vi "XLP80_Action_InitControls.vi"(8 "err in":errorcluster) -> (0 "err out":errorcluster)   [LabVIEW 2021]
uses:
  XLP80_General_Libs/WL_Libs_V14.25/WL_Alarm_V14.00.llb/WL_Alarm_TypeDefClusterStatus.ctl
  XLP80_GUI_V001.llb/XLP80_GUI_TDefEnumMessages.ctl
  XLP80_HH/XLP80_HH_TDefsCluster_HH Setpoint.ctl
  XLP80_Globals/Globals_Settings_XLP80.vi
  XLP80_Globals/XLP80_Globals_Status.vi
  XLP80_Globals/XLP80_Globals_Referenzen.vi
  XLP80_Datalog/XLP80_Datalog_Globals.vi
  XLP80_Alarm_V001.llb/XLP80_Alarm_Globals.vi
  XLP80_HH/XLP80_HH_Globals.vi
  XLP80_General_Libs/WL_Libs_V14.25/WL_Alarm_V14.00.llb/WL_Alarm_Globals.vi
  XLP80_Auto_V001.llb/XLP80_Auto_Globals.vi
  XLP80_General_Libs/WL_Libs_V14.25/WL_Profile_V14.00.llb/WL_Profile_Globals.vi
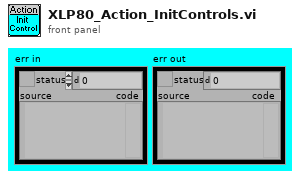
[diagram p1: front panel]
types:
  T1 = typedef "XLP80_Action_TDefEnumControl.ctl" = enum16{"Testmode_A", "Testmode_B"}
  T2 = cluster{"Comment":string, "SamplingRate":u32, "Logging":bool, "FileName":string}
  T3 = enum32{"Debug", "CAN", "Testbench", "Load", "CVM", "P&ID", "Datalog"}
  T4 = enum32{"Debug", "P&ID", "I/Os", "Regulator", "Datalog", "Automatic", "Load", "Charts", "CVM"}
  T5 = typedef "XLP80_GUI_TDefEnumMessages.ctl" = enum16{"Clear", "Add"}
  T6 = typedef "XLP80_HH_TDefsCluster_HH Setpoint.ctl" = cluster{"Enable Input":bool, "Set Current":sgl, "Set Voltage":sgl, "Set Power":sgl}
  T7 = typedef "WL_Alarm_TypeDefClusterStatus.ctl" = cluster{"NOTAUS":bool, "ABSCHALTEN":bool, "MELDUNG":bool}
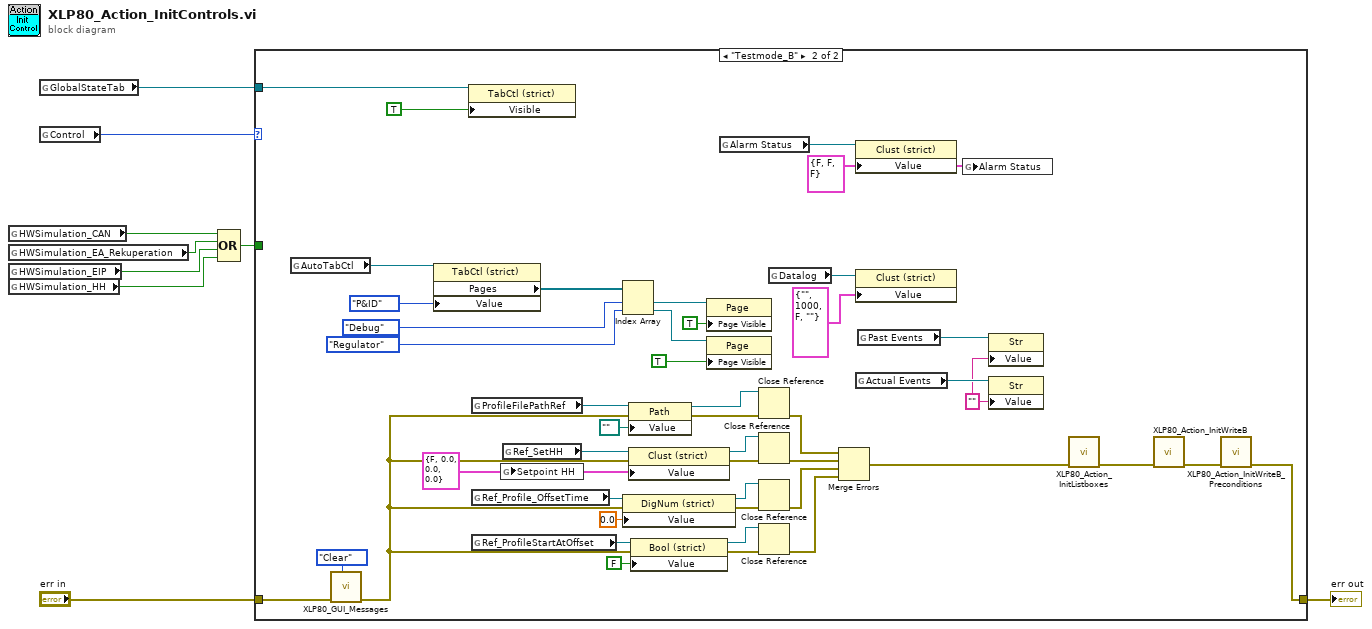
[diagram p0: block diagram]
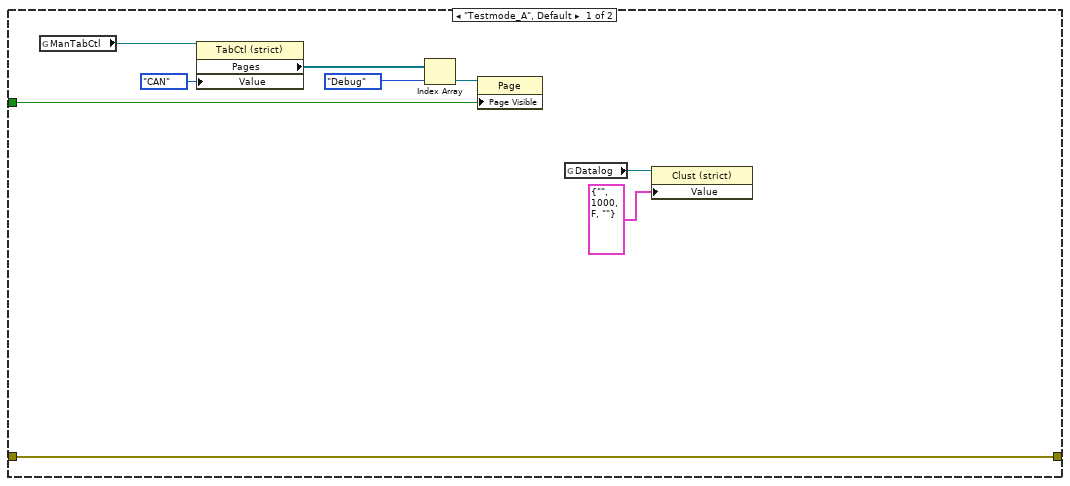
[diagram p2: hidden frame]
diagram:
  n1 = global read "Globals_Settings_XLP80.vi" "HWSimulation_CAN"() -> (w5:bool)
  n2 = global read "Globals_Settings_XLP80.vi" "HWSimulation_EA_Rekuperation"() -> (w4:bool)
  n3 = global read "Globals_Settings_XLP80.vi" "HWSimulation_EIP"() -> (w3:bool)
  n4 = global read "Globals_Settings_XLP80.vi" "HWSimulation_HH"() -> (w2:bool)
  n5 = global read "XLP80_Globals_Referenzen.vi" "GlobalStateTab"() -> (w6:refnum<vi>)
  n6 = global read "XLP80_Globals_Status.vi" "Control"() -> (w7:T1)
  n7 = Compound Arithmetic op=OR(w5, w4, w3, w2) -> (w1:bool)
  n8 = case shown="\"Testmode_B\"" w7 {
    tunnel: "err in" -> [w12 w63]
    tunnel: w1 -> [w15 _]
    tunnel: [w12 w22] -> w8
    tunnel: w6 -> [_ w52]
    frame "Testmode_A", Default {
      n9 = global read "XLP80_Globals_Referenzen.vi" "ManTabCtl"() -> (w18:refnum<vi>)
      n10 = property class="TabCtl (strict)"(reference=w18, "Value"=T3."CAN") -> ("Pages"=w17:refnum<vi>[])  [unwired: 1 in, 2 out]
      n11 = Index Array(array=w17, index=T3."Debug" ("Value")) -> (element=w16:refnum<vi>)
      n12 = property class="Page"(reference=w16, "Page Visible"=w15) -> ()  [unwired: 1 in, 2 out]
      n13 = global read "XLP80_Datalog_Globals.vi" "Datalog"() -> (w10:refnum<vi>)
      n14 = property class="Clust (strict)"(reference=w10, "Value"=T2 {"Comment"="", "SamplingRate"=1000, "Logging"=FALSE, "FileName"=""}) -> ()  [unwired: 1 in, 2 out]
    }
    frame "Testmode_B" {
      w24 = T6 {"Enable Input"=FALSE, "Set Current"=0.0, "Set Voltage"=0.0, "Set Power"=0.0} ("Value")
      w58 = T7 {"NOTAUS"=FALSE, "ABSCHALTEN"=FALSE, "MELDUNG"=FALSE} ("Alarm Status")
      w55 = "" ("Value")
      n15 = global read "XLP80_Globals_Referenzen.vi" "AutoTabCtl"() -> (w62:refnum<vi>)
      n16 = call "XLP80_GUI_Messages.vi"("Message"=XLP80_GUI_TDefEnumMessages."Clear", "err in"=w63) -> ("err out"=w27:errorcluster)  [unwired: 9 in]
      n17 = property class="TabCtl (strict)"(reference=w62, "Value"=T4."P&ID") -> ("Pages"=w61:refnum<vi>[])  [unwired: 1 in, 2 out]
      n18 = property class="TabCtl (strict)"(reference=w52, "Visible"=TRUE) -> ()  [unwired: 1 in, 2 out]
      n19 = global read "WL_Profile_Globals.vi" "ProfileFilePathRef"() -> (w41:refnum<vi>)
      n20 = global read "XLP80_Auto_Globals.vi" "Ref_Profile_OffsetTime"() -> (w33:refnum<vi>)
      n21 = global read "XLP80_Auto_Globals.vi" "Ref_ProfileStartAtOffset"() -> (w31:refnum<vi>)
      n22 = global write "XLP80_HH_Globals.vi" "Setpoint HH"(w24) -> ()
      n23 = global read "XLP80_Auto_Globals.vi" "Ref_SetHH"() -> (w46:refnum<vi>)
      n24 = Index Array(array=w61, index #1=T4."Debug" ("Value"), index #2=T4."Regulator" ("Value")) -> (element #1=w60:refnum<vi>, element #2=w49:refnum<vi>)
      n25 = property class="DigNum (strict)"(reference=w33, error in=w27, "Value"=sgl 0.0) -> (reference out=w37:refnum<vi>, error out=w36:errorcluster)
      n26 = property class="Path"(reference=w41, error in=w27, "Value"=path "") -> (reference out=w39:refnum<vi>, error out=w40:errorcluster)
      n27 = property class="Clust (strict)"(reference=w46, error in=w27, "Value"=w24) -> (reference out=w44:refnum<vi>, error out=w45:errorcluster)
      n28 = property class="Bool (strict)"(reference=w31, error in=w27, "Value"=FALSE) -> (reference out=w34:refnum<vi>, error out=w35:errorcluster)
      n29 = property class="Page"(reference=w60, "Page Visible"=TRUE) -> ()  [unwired: 1 in, 2 out]
      n30 = property class="Page"(reference=w49, "Page Visible"=TRUE) -> ()  [unwired: 1 in, 2 out]
      n31 = global read "WL_Alarm_Globals.vi" "Alarm Status"() -> (w59:refnum<vi>)
      n32 = Close Reference(reference=w39, error in (no error)=w40) -> (error out=w38:errorcluster)
      n33 = Close Reference(reference=w44, error in (no error)=w45) -> (error out=w43:errorcluster)
      n34 = Close Reference(reference=w37, error in (no error)=w36) -> (error out=w29:errorcluster)
      n35 = Close Reference(reference=w34, error in (no error)=w35) -> (error out=w28:errorcluster)
      n36 = global read "XLP80_Datalog_Globals.vi" "Datalog"() -> (w54:refnum<vi>)
      n37 = Merge Errors(w38, w43, w29, w28) -> (w26:errorcluster)
      n38 = property class="Clust (strict)"(reference=w59, "Value"=w58) -> ()  [unwired: 1 in, 2 out]
      n39 = property class="Clust (strict)"(reference=w54, "Value"=T2 {"Comment"="", "SamplingRate"=1000, "Logging"=FALSE, "FileName"=""}) -> ()  [unwired: 1 in, 2 out]
      n40 = global read "WL_Alarm_Globals.vi" "Actual Events"() -> (w56:refnum<vi>)
      n41 = global read "WL_Alarm_Globals.vi" "Past Events"() -> (w57:refnum<vi>)
      n42 = global write "XLP80_Alarm_Globals.vi" "Alarm Status"(w58) -> ()
      n43 = property class="Str"(reference=w57, "Value"=w55) -> ()  [unwired: 1 in, 2 out]
      n44 = property class="Str"(reference=w56, "Value"=w55) -> ()  [unwired: 1 in, 2 out]
      n45 = call "XLP80_Action_InitListboxes.vi"("err in"=w26) -> ("err out"=w25:errorcluster)  [unwired: 10 in]
      n46 = call "XLP80_Action_InitWriteB.vi"("err in"=w25) -> ("err out"=w23:errorcluster)  [unwired: 10 in]
      n47 = call "XLP80_Action_InitWriteB_Preconditions.vi"("err in"=w23) -> ("err out"=w22:errorcluster)  [unwired: 10 in]
    }
  }
  "err out" <- w8
